vi "Offset_remover.vi"(1 "threshold Peaks":dbl format="%0.2f", 2 "Graphe":waveform(dbl)) -> (0 "waveform out":waveform(dbl))   [LabVIEW 2023]
uses:
  <vilib>/Analysis/baseanly.llb/Mean (DBL).vi
  <vilib>/Analysis/NI_AALBase.lvlib
  <vilib>/Analysis/NI_AAL_SigProc.lvlib
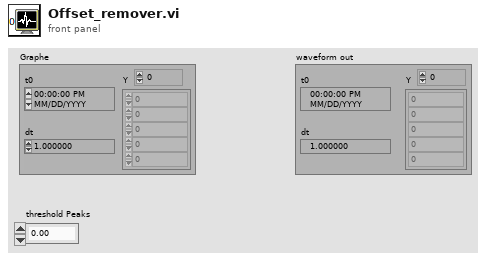
[diagram p1: front panel]
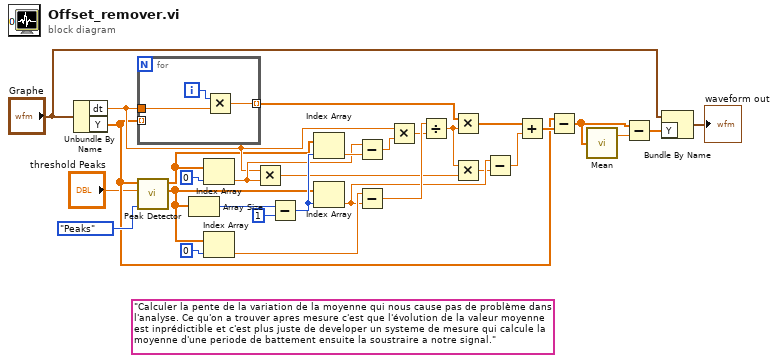
[diagram p0: block diagram]
diagram:
  (unwired) "Calculer la pente de la variation de la moyenne qui nous cause pas de problème dans l'analyse. Ce qu'on a trouver apres mesure c'est que l'évolution de la valeur moyenne est inprédictible et c'est plus juste de developer un systeme de mesure qui calcule la moyenne d'une periode de battement ensuite la soustraire a notre signal."
  n1 = Unbundle By Name("Graphe") -> ("dt"=w5:dbl, "Y"=w2:dbl[])
  n2 = for {
    tunnel: w5 -> [w32]
    tunnel: [w31] -> w16 mode=indexing
    tunnel: w2 -> [_] mode=indexing
    i -> [w33]
    n3 = Multiply(x=w33, y=w32) -> (x*y=w31:dbl)
  }
  n4 = call <vilib>:"Peak Detector.vi"("peaks/valleys"=enum32{"Peaks", "Valleys"}."Peaks", "threshold"="threshold Peaks", "X"=w2) -> ("Amplitudes"=w4:dbl[], "Locations"=w3:dbl[])  [unwired: 4 in, 3 out]
  n5 = Array Size(array=w4) -> (size(s)=w25:i32)
  n6 = Index Array(array=w3, index=0) -> (element=w12:dbl)
  n7 = Index Array(array=w4, index=0) -> (element=w27:dbl)
  n8 = Multiply(x=w5, y=w12) -> (x*y=w13:dbl)
  n9 = Subtract(x=w25, y=1) -> (x-y=w23:i32)
  n10 = Index Array(array=w3, index=w23) -> (element=w22:dbl)
  n11 = Index Array(array=w4, index=w23) -> (element=w19:dbl)
  n12 = Subtract(x=w12, y=w22) -> (x-y=w14:dbl)
  n13 = Subtract(x=w27, y=w19) -> (x-y=w28:dbl)
  n14 = Multiply(x=w5, y=w14) -> (x*y=w15:dbl)
  n15 = Divide(x=w28, y=w15) -> (x/y=w20:dbl)
  n16 = Multiply(x=w16, y=w20) -> (x*y=w21:dbl[])
  n17 = Multiply(x=w20, y=w13) -> (x*y=w18:dbl)
  n18 = Subtract(x=w19, y=w18) -> (x-y=w17:dbl)
  n19 = Add(x=w21, y=w17) -> (x+y=w29:dbl[])
  n20 = Subtract(x=w2, y=w29) -> (x-y=w10:dbl[])
  n21 = call-poly <vilib>:"Mean.vi"("X"=w10) -> ("mean"=w9:dbl)  [unwired: 1 out]
  n22 = Subtract(x=w10, y=w9) -> (x-y=w8:dbl[])
  n23 = Bundle By Name(cluster="Graphe", "Y"=w8) -> (→"waveform out":waveform(dbl))
